vi "(자동)gugudan server.vi"() -> ()   [LabVIEW 2014]
uses:
  <vilib>/FTP/NI_FTP.lvlib
panel:
  in  "address 2":string="ip address"
  out "Client ip address":string="Client ip address"
  in  "사용설명서":bool
  out "로그인":bool
  in  "ID":string="ID"
  in  "PW":string="PW"
  in  "E-Mail":string="E-Mail  address"
  in  "명령전달":bool
  out "명령코드":i16[](array[numeric])
  out "참 거짓":string="상태창입니다."
  out "문자열":string="명령창 입니다."
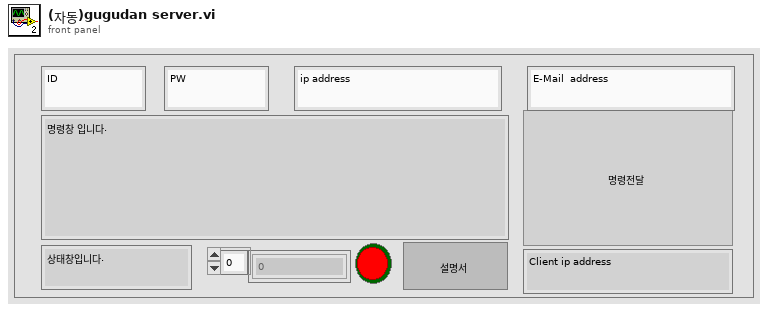
[diagram p1: front panel]
types:
  T1 = typedef "NI_FTP.lvlib/FTP Session.ctl" = refnum<k5>
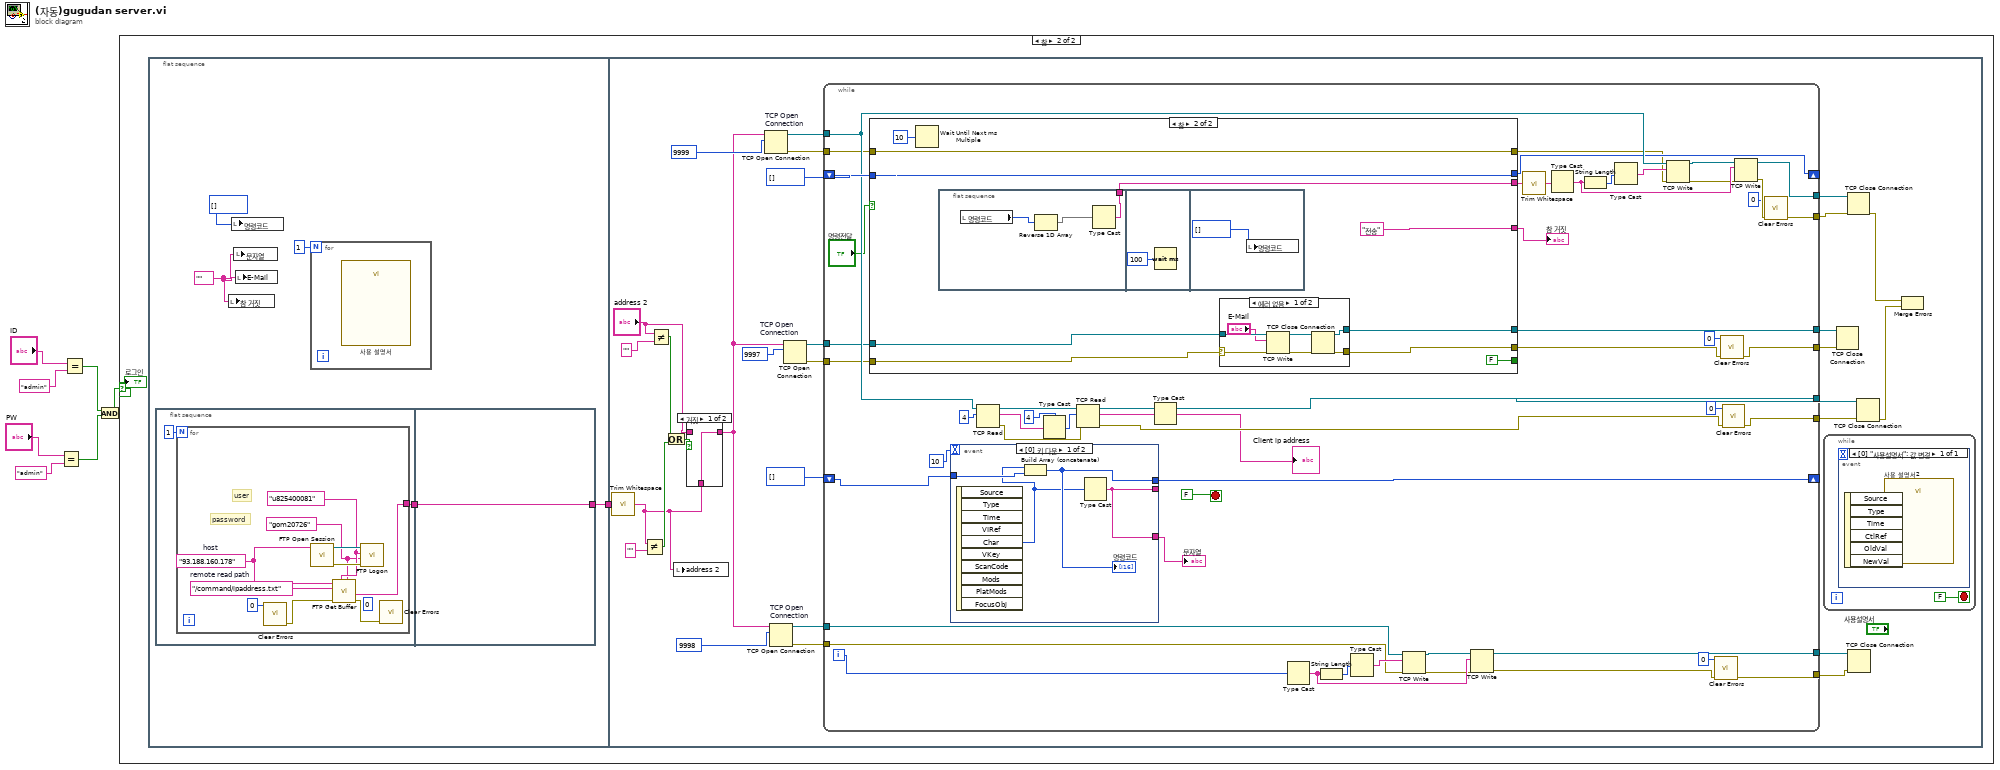
[diagram p0: block diagram]
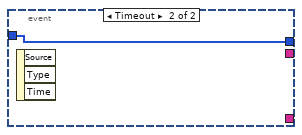
[diagram p4: hidden frame]
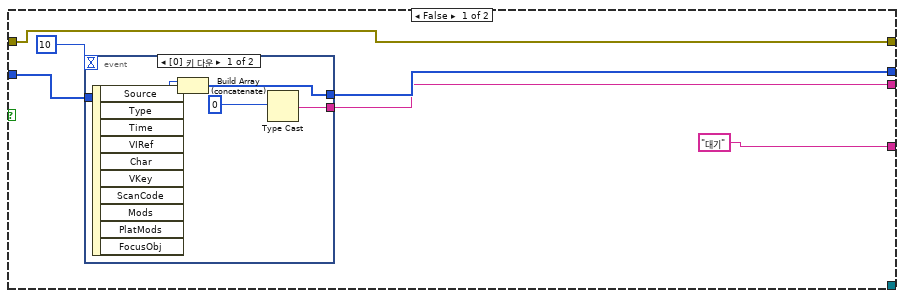
[diagram p5: hidden frame]
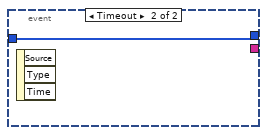
[diagram p6: hidden frame]
diagram:
  n1 = Equal?(x="PW", y="admin") -> (x = y?=w2:bool)
  n2 = Equal?(x="ID", y="admin") -> (x = y?=w3:bool)
  n3 = And(x=w3, y=w2) -> (x .and. y?=w1:bool)
  n4 = case shown="참" w1 {
    selector: w1 -> [_ w9]
    frame False {
    }
    frame True {
      n5 = flat-sequence {
        tunnel: [w10] -> w8
        tunnel: w8 -> [w36]
        frame #0 {
          w13 = ""
          n6 = flat-sequence {
            tunnel: [w16] -> w11
            tunnel: [w27] -> w10
            tunnel: w11 -> [w27]
            frame #0 {
              n7 = for {
                N: 1 -> [_]
                tunnel: [w20] -> w16
                (unwired) 0 ("specific error code to clear (0: all)")
                w23 = "gom20726"
                w24 = "u825400081"
                w21 = "/command/ipaddress.txt"  # remote read path
                w22 = "93.188.160.178"  # host
                # "user"
                # "password"
                n8 = call <vilib>:"Clear Errors.vi"("specific error code to clear (0: all)"=0) -> ("error out"=w19:errorcluster)  [unwired: 5 in, 1 out]
                n9 = call <vilib>:"FTP Open Session.vi"("address"=w22) -> ("error out"=w25:errorcluster, "ftp session"=w26:T1)  [unwired: 7 in, 2 out]
                n10 = call <vilib>:"FTP Get Buffer.vi"("password"=w23, "user"=w24, "error in (no error)"=w19, "remote path"=w21, "host"=w22) -> ("error out"=w17:errorcluster, "data"=w20:string)  [unwired: 4 in, 1 out]
                n11 = call <vilib>:"FTP Logon.vi"("error in (no error)"=w25, "password"=w23, "user"=w24, "ftp session"=w26) -> ()  [unwired: 4 in, 4 out]
                n12 = call <vilib>:"Clear Errors.vi"("error in (no error)"=w17) -> ()  [unwired: 5 in, 2 out]
              }
            }
            frame #1 {
            }
          }
          n13 = local write "참 거짓"(w13) -> ()
          n14 = local write "명령코드"(i16[] []) -> ()
          n15 = local write "문자열"(w13) -> ()
          n16 = local write "E-Mail"(w13) -> ()
          n17 = for {
            N: 1 -> [_]
            n18 = call "사용 설명서"() -> ()  [unwired: 10 in, 2 out]
          }
        }
        frame #1 {
          n19 = call <vilib>:"Trim Whitespace.vi"("string"=w36) -> ("trimmed string"=w29:string)  [unwired: 1 in]
          n20 = Not Equal?(x=w29, y="") -> (x != y?=w32:bool)
          n21 = Not Equal?(x="address 2", y="") -> (x != y?=w33:bool)
          n22 = Or(x=w33, y=w32) -> (x .or. y?=w31:bool)
          n23 = local write "address 2"(w29) -> ()
          n24 = case shown="거짓" w31 {
            tunnel: "address 2" -> [_ w59]
            tunnel: w29 -> [w58 _]
            tunnel: [w58 w59] -> w28
            frame False {
            }
            frame True {
            }
          }
          n25 = TCP Open Connection "TCP Open \nConnection"(address=w28, remote port or service name=u16 9999) -> (connection ID=w57:refnum<k5>, error out=w51:errorcluster)  [unwired: 3 in]
          n26 = TCP Open Connection "TCP Open \nConnection"(address=w28, remote port or service name=u16 9998) -> (connection ID=w46:refnum<k5>, error out=w43:errorcluster)  [unwired: 3 in]
          n27 = TCP Open Connection "TCP Open \nConnection"(address=w28, remote port or service name=u16 9997 ("원격 포트 또는 서비스 이름")) -> (connection ID=w41:refnum<k5>, error out=w40:errorcluster)  [unwired: 3 in]
          n28 = while {
            tunnel: w57 -> [w106]
            tunnel: [w113] -> w55
            shift-right: [w95] -> _
            shift-left: i16[] [] -> [w112]
            tunnel: [w105] -> w54
            shift-right: [w96] -> _
            shift-left: i16[] [] -> [w97]
            tunnel: w51 -> [w94]
            tunnel: [w73] -> w37
            tunnel: [w70] -> w49
            tunnel: w46 -> [w81]
            tunnel: [w80] -> w45
            tunnel: [w68] -> w44
            tunnel: w43 -> [w79]
            tunnel: [w64] -> w42
            tunnel: w41 -> [w77]
            tunnel: w40 -> [w76]
            tunnel: [w75] -> w38
            i -> [w78]
            stop <- FALSE stop-if-true
            n29 = case shown="참" "명령전달" {
              tunnel: w112 -> [w124 w140]
              tunnel: [w123 w140] -> w95
              tunnel: [w121 w136] -> w89
              tunnel: w94 -> [w120 w138]
              tunnel: [w120 w138] -> w93
              tunnel: ["대기" "전송"] -> w88
              tunnel: [_ FALSE ("불리언")] -> _
              tunnel: [_ w134] -> w63
              tunnel: w77 -> [_ w133]
              tunnel: w76 -> [_ w132]
              tunnel: [_ w131] -> w75
              frame False {
                n30 = event shown="[0] 키 다운" {
                  selector: _ -> [_ _]
                  dyn-events: _ -> [_ _]
                  timeout: 10 -> [_ _]
                  tunnel: [w128 w130] -> w123
                  tunnel: w124 -> [w129 w130]
                  tunnel: [w126 _] -> w121
                  event Key Down {
                    n31 = event-data() -> ("Char"=w127:i16)  [unwired: 1 in, 9 out]
                    n32 = Build Array (concatenate)(w127, w129) -> (w128:i16[])
                    n33 = Type Cast(x=0) -> (*(type *) &x=w126:string)  [unwired: 1 in]
                  }
                  event Timeout {
                    n34 = event-data() -> ()  [unwired: 1 in, 3 out]
                  }
                }
              }
              frame True {
                n35 = Wait Until Next ms Multiple(millisecond multiple=u32 10) -> ()  [unwired: 1 out]
                n36 = flat-sequence {
                  tunnel: [w151] -> w136
                  frame #0 {
                    n37 = local read "명령코드"() -> (w152:i16[])
                    n38 = Reverse 1D Array(array=w152) -> (reversed array=w150:i16[])
                    n39 = Type Cast(x=w150) -> (*(type *) &x=w151:string)  [unwired: 1 in]
                  }
                  frame #1 {
                    n40 = Wait (ms)(milliseconds to wait=u32 100 ("대기 시간(ms)")) -> ()  [unwired: 1 out]
                  }
                  frame #2 {
                    n41 = local write "명령코드"(i16[] []) -> ()
                  }
                }
                n42 = case shown="에러 없음" w132 {
                  selector: w132 -> [w142 w149]
                  tunnel: [w146 w148] -> w131
                  tunnel: [w145 w149] -> w134
                  tunnel: w133 -> [w143 w148]
                  frame No Error {
                    n43 = TCP Write(connection ID=w143, data in="E-Mail", error in (no error)=w142) -> (connection ID out=w147:refnum<k5>, error out=w144:errorcluster)  [unwired: 2 out]
                    n44 = TCP Close Connection(connection ID=w147, error in (no error)=w144) -> (connection ID out=w146:refnum<k5>, error out=w145:errorcluster)  [unwired: 1 out]
                  }
                  frame Error {
                  }
                }
              }
            }
            "참 거짓" <- w88
            n45 = event shown="[0] 키 다운" {
              selector: _ -> [_ _]
              dyn-events: _ -> [_ _]
              timeout: 10 -> [_ _]
              tunnel: [w115 w118] -> w96
              tunnel: [w117 _] -> w98
              tunnel: [w117 _] -> _
              tunnel: w97 -> [w116 w118]
              event Key Down {
                n46 = event-data() -> ("Char"=w114:i16)  [unwired: 1 in, 9 out]
                n47 = Build Array (concatenate)(w114, w116) -> (w115:i16[])
                "명령코드" <- w115
                n48 = Type Cast(x=w114) -> (*(type *) &x=w117:string)  [unwired: 1 in]
              }
              event Timeout {
                n49 = event-data() -> ()  [unwired: 1 in, 3 out]
              }
            }
            "문자열" <- w98
            n50 = TCP Read(connection ID=w106, bytes to read=4) -> (connection ID out=w111:refnum<k5>, data out=w109:string, error out=w91:errorcluster)  [unwired: 3 in]
            n51 = Type Cast(type=4 ("bytes to read"), x=w109) -> (*(type *) &x=w108:i32)
            n52 = TCP Read(connection ID=w111, bytes to read=w108, error in (no error)=w91) -> (connection ID out=w105:refnum<k5>, data out=w107:string, error out=w69:errorcluster)  [unwired: 2 in]
            n53 = Type Cast(x=w107) -> (*(type *) &x=→"Client ip address":string)  [unwired: 1 in]
            n54 = Type Cast(x=w78) -> (*(type *) &x=w83:string)  [unwired: 1 in]
            n55 = String Length(string=w83) -> (length=w84:i32)
            n56 = Type Cast(x=w84) -> (*(type *) &x=w85:string)  [unwired: 1 in]
            n57 = TCP Write(connection ID=w81, data in=w85, error in (no error)=w79) -> (connection ID out=w86:refnum<k5>, error out=w82:errorcluster)  [unwired: 1 in, 1 out]
            n58 = TCP Write(connection ID=w86, data in=w83, error in (no error)=w82) -> (connection ID out=w80:refnum<k5>, error out=w67:errorcluster)  [unwired: 1 in, 1 out]
            n59 = call <vilib>:"Trim Whitespace.vi"("string"=w89) -> ("trimmed string"=w90:string)  [unwired: 1 in]
            n60 = Type Cast(x=w90) -> (*(type *) &x=w100:string)  [unwired: 1 in]
            n61 = String Length(string=w100) -> (length=w101:i32)
            n62 = Type Cast(x=w101) -> (*(type *) &x=w102:string)  [unwired: 1 in]
            n63 = TCP Write(connection ID=w106, data in=w102, error in (no error)=w93) -> (connection ID out=w103:refnum<k5>, error out=w92:errorcluster)  [unwired: 1 in, 1 out]
            n64 = call <vilib>:"Clear Errors.vi"("error in (no error)"=w67, "specific error code to clear (0: all)"=0) -> ("error out"=w68:errorcluster)  [unwired: 4 in, 1 out]
            n65 = call <vilib>:"Clear Errors.vi"("error in (no error)"=w63, "specific error code to clear (0: all)"=0) -> ("error out"=w64:errorcluster)  [unwired: 4 in, 1 out]
            n66 = call <vilib>:"Clear Errors.vi"("error in (no error)"=w69, "specific error code to clear (0: all)"=0) -> ("error out"=w70:errorcluster)  [unwired: 4 in, 1 out]
            n67 = TCP Write(connection ID=w103, data in=w100, error in (no error)=w92) -> (connection ID out=w113:refnum<k5>, error out=w72:errorcluster)  [unwired: 1 in, 1 out]
            n68 = call <vilib>:"Clear Errors.vi"("error in (no error)"=w72, "specific error code to clear (0: all)"=0) -> ("error out"=w73:errorcluster)  [unwired: 4 in, 1 out]
          }
          n69 = while {
            stop <- FALSE stop-if-true
            n70 = event shown="[0] \"사용설명서\": 값 변경" {
              selector: _ -> [_]
              dyn-events: _ -> [_]
              timeout: _ -> [_]
              event "사용설명서": Value Change {
                n71 = event-data() -> ()  [unwired: 1 in, 6 out]
                n72 = call "사용 설명서2"() -> ()  [unwired: 10 in, 2 out]
              }
            }
          }
          n73 = TCP Close Connection(connection ID=w38, error in (no error)=w42) -> ()  [unwired: 3 out]
          n74 = TCP Close Connection(connection ID=w55, error in (no error)=w37) -> (error out=w50:errorcluster)  [unwired: 1 in, 1 out]
          n75 = TCP Close Connection(connection ID=w45, error in (no error)=w44) -> ()  [unwired: 1 in, 2 out]
          n76 = TCP Close Connection(connection ID=w54, error in (no error)=w49) -> (error out=w48:errorcluster)  [unwired: 1 in, 1 out]
          n77 = Merge Errors(w50, w48) -> ()  [unwired: 1 out]
        }
      }
      "로그인" <- w9
    }
  }
